vi "mainActivity_关闭模块的消息簇.vi"(1 "模块注册信息":T1) -> (0 "消息簇":cluster{"相对路径":string, "相对路径":string})   [LabVIEW 2014]
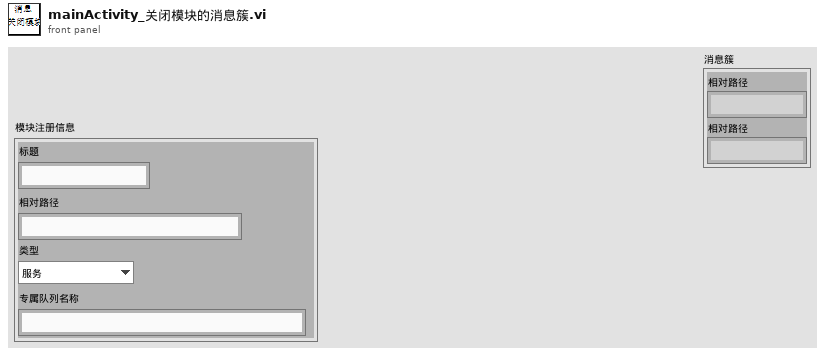
[diagram p1: front panel]
types:
  T1 = cluster{"标题":string, "相对路径":string, "类型":enum16{"服务", "活动"}, "专属队列名称":string}
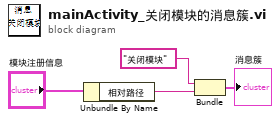
[diagram p0: block diagram]
diagram:
  n1 = Unbundle By Name("模块注册信息") -> ("相对路径"=w3:string)
  n2 = Bundle("相对路径"="关闭模块", "相对路径"=w3) -> (→"消息簇":cluster{"相对路径":string, "相对路径":string})  [unwired: 1 in]
